vi "ReverseWaveforms.vi"(11 "signals in":waveform(dbl)[](array[waveform])) -> (3 "signals out":waveform(dbl)[](array[waveform]))   [LabVIEW 2015]
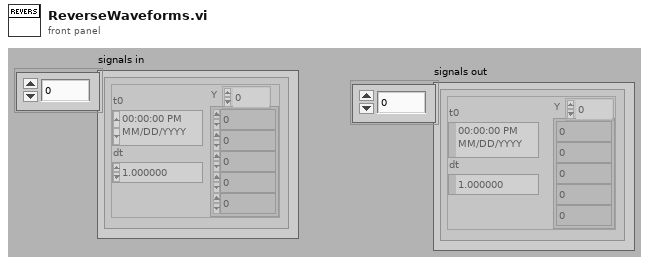
[diagram p1: front panel]
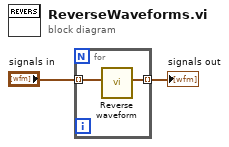
[diagram p0: block diagram]
diagram:
  n1 = for {
    tunnel: "signals in" -> [w4] mode=indexing
    tunnel: [w3] -> w1 mode=indexing
    n2 = call "Reverse waveform.vi"("Waveform"=w4) -> ("Output Waveform"=w3:waveform(dbl))  [unwired: 10 in]
  }
  "signals out" <- w1
